vi "Execute_Circle_v3.vi"(0 "x-disp inp.":sgl[](array[numeric]), 1 "y-disp inp.":sgl[](array[numeric]), 2 "Resolution":u16=20, 3 "Speed":i32=200, 4 "Current (mA)":dbl, 5 "Laser GPIB":u8=10 max=100, 6 "Motor GPIB":u8=6) -> ()   [LabVIEW 2010]
uses:
  <vilib>/express/express arith-compare/Formula/XNode/ExpressFormulaBlockNode.xnode
panel:
  out "Dummy":string
  out "y-speed":sgl
  out "y-dist":sgl
  out "y-LR":bool
  out "x-speed":sgl
  out "x-dist":sgl
  out "x-LR":bool=TRUE
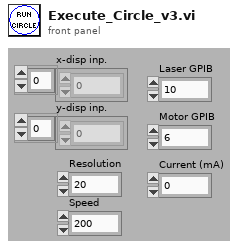
[diagram p1: front panel]
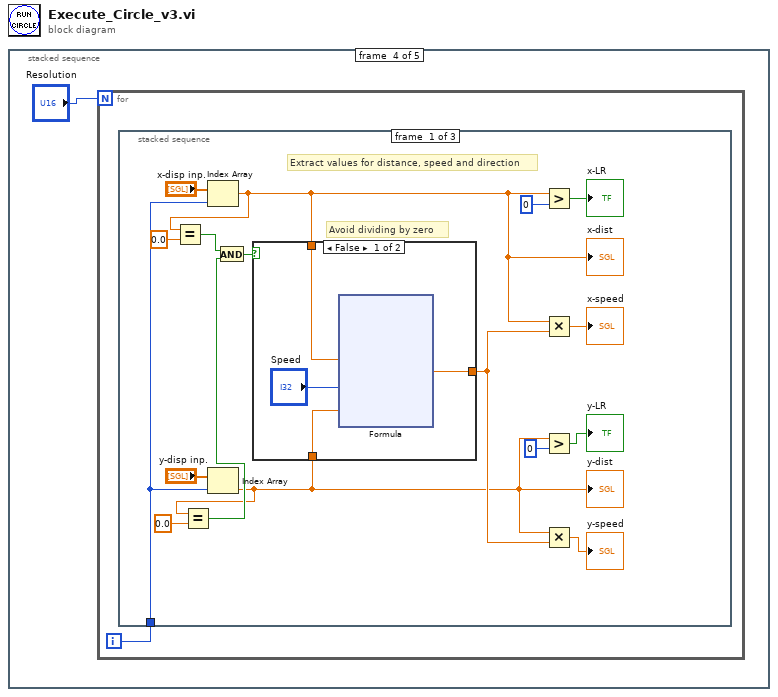
[diagram p0: block diagram]
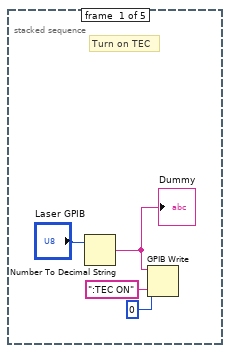
[diagram p2: hidden frame]
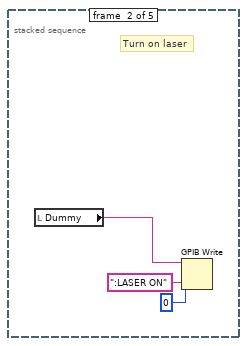
[diagram p3: hidden frame]
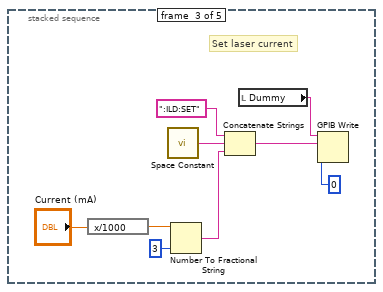
[diagram p4: hidden frame]
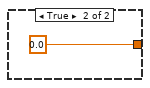
[diagram p5: hidden frame]
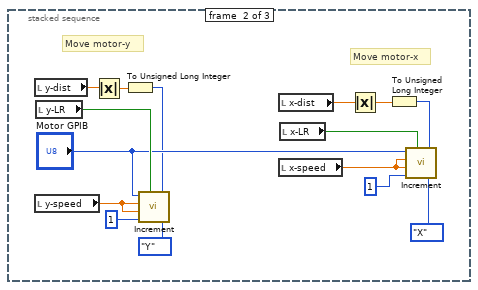
[diagram p6: hidden frame]
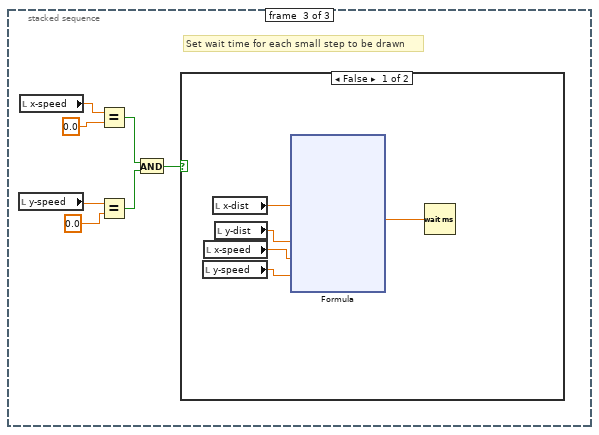
[diagram p7: hidden frame]
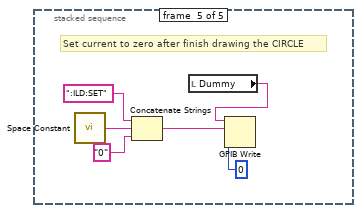
[diagram p9: hidden frame]
diagram:
  n1 = stacked-sequence {
    frame #0 {
      # "Turn on TEC"
      n2 = Number To Decimal String(number="Laser GPIB") -> (decimal integer string=w1:string)  [unwired: 1 in]
      "Dummy" <- w1
      n3 = GPIB Write(0:w1, 1:":TEC ON" ("data"), 2:i16 0 ("mode (0)")) -> ()  [unwired: 2 in, 2 out]
    }
    frame #1 {
      # "Turn on laser"
      n4 = local read "Dummy"() -> (w5:string)
      n5 = GPIB Write(0:w5, 1:":LASER ON" ("data"), 2:i16 0 ("mode (0)")) -> ()  [unwired: 2 in, 2 out]
    }
    frame #2 {
      # "Set laser current"
      n6 = expression code="x/1000"("Current (mA)") -> (w12:dbl)
      n7 = call <vilib>:"Space Constant.vi"() -> ("String"=w14:string)
      n8 = Number To Fractional String(number=w12, precision (6)=i16 3) -> (F-format string=w9:string)  [unwired: 2 in]
      n9 = Concatenate Strings(":ILD:SET", w14, w9) -> (w13:string)
      n10 = local read "Dummy"() -> (w8:string)
      n11 = GPIB Write(0:w8, 1:w13, 2:i16 0 ("mode (0)")) -> ()  [unwired: 2 in, 2 out]
    }
    frame #3 {
      n12 = for {
        N: "Resolution" -> [_]
        i -> [w18]
        n13 = stacked-sequence {
          tunnel: w18 -> [w33 _ _]
          frame #0 {
            # "Extract values for distance, speed and direction"
            # "Avoid dividing by zero"
            n14 = Index Array(array="x-disp inp.", index=w33) -> (element=w22:sgl)
            "x-dist" <- w22
            n15 = Equal?(x=w22, y=sgl 0.0) -> (x = y?=w30:bool)
            n16 = Index Array(array="y-disp inp.", index=w33) -> (element=w20:sgl)
            "y-dist" <- w20
            n17 = Equal?(x=w20, y=sgl 0.0) -> (x = y?=w29:bool)
            n18 = And(x=w30, y=w29) -> (x .and. y?=w28:bool)
            n19 = case shown="False" w28 {
              tunnel: [w36 sgl 0.0] -> w27
              tunnel: w22 -> [w38 _]
              tunnel: w20 -> [w37 _]
              frame False {
                n20 = xnode "Formula"("X1"=w38, "X2"="Speed", "X3"=w37) -> ("Result"=w36:sgl)  [unwired: 1 in, 1 out]
              }
              frame True {
              }
            }
            n21 = Greater?(x=w22, y=i8 0) -> (0:→"x-LR":bool)
            n22 = Multiply(x=w22, y=w27) -> (x*y=→"x-speed":sgl)
            n23 = Greater?(x=w20, y=i8 0) -> (0:→"y-LR":bool)
            n24 = Multiply(x=w20, y=w27) -> (x*y=→"y-speed":sgl)
          }
          frame #1 {
            # "Move motor-x"
            # "Move motor-y"
            n25 = local read "y-dist"() -> (w57:sgl)
            n26 = local read "y-speed"() -> (w65:sgl)
            n27 = local read "y-LR"() -> (w64:bool)
            n28 = Absolute Value(x=w57) -> (abs(x)=w58:sgl)
            n29 = To Unsigned Long Integer(number=w58) -> (unsigned 32bit integer=w55:u32)
            n30 = call "Increment.vi"("GPIB_Addr"="Motor GPIB", "F Speed"=w65, "L Speed"=w65, "Rate"=u16 1, "CCW 3"=w64, "Distance"=w55, "Axis"=enum16{"X", "Y", "Z", "U", "V", "W"}."Y") -> ()
            n31 = local read "x-dist"() -> (w54:sgl)
            n32 = local read "x-speed"() -> (w60:sgl)
            n33 = local read "x-LR"() -> (w61:bool)
            n34 = Absolute Value(x=w54) -> (abs(x)=w56:sgl)
            n35 = To Unsigned Long Integer(number=w56) -> (unsigned 32bit integer=w53:u32)
            n36 = call "Increment.vi"("GPIB_Addr"="Motor GPIB", "F Speed"=w60, "L Speed"=w60, "Rate"=u16 1, "CCW 3"=w61, "Distance"=w53, "Axis"=enum16{"X", "Y", "Z", "U", "V", "W"}."X") -> ()
          }
          frame #2 {
            # "Set wait time for each small step to be drawn"
            n37 = local read "y-speed"() -> (w72:sgl)
            n38 = local read "x-speed"() -> (w74:sgl)
            n39 = Equal?(x=w74, y=sgl 0.0) -> (x = y?=w70:bool)
            n40 = Equal?(x=w72, y=sgl 0.0) -> (x = y?=w69:bool)
            n41 = And(x=w70, y=w69) -> (x .and. y?=w68:bool)
            n42 = case shown="False" w68 {
              frame False {
                n43 = local read "y-speed"() -> (w76:sgl)
                n44 = local read "x-speed"() -> (w78:sgl)
                n45 = local read "x-dist"() -> (w79:sgl)
                n46 = local read "y-dist"() -> (w77:sgl)
                n47 = xnode "Formula"("X1"=w79, "X2"=w77, "X3"=w78, "X4"=w76) -> ("Result"=w75:sgl)  [unwired: 1 in, 1 out]
                n48 = Wait (ms)(milliseconds to wait=w75) -> ()  [unwired: 1 out]
              }
              frame True {
              }
            }
          }
        }
      }
    }
    frame #4 {
      # "Set current to zero after finish drawing the CIRCLE"
      n49 = call <vilib>:"Space Constant.vi"() -> ("String"=w96:string)
      n50 = Concatenate Strings(":ILD:SET", w96, "0" ("string")) -> (w97:string)
      n51 = local read "Dummy"() -> (w98:string)
      n52 = GPIB Write(0:w98, 1:w97, 2:i16 0 ("mode (0)")) -> ()  [unwired: 2 in, 2 out]
    }
  }
